vi "initial-Pos-Z.vi"(8 "error in (no error)":errorcluster) -> (0 "error out":errorcluster, 3 "Z position":dbl)   [LabVIEW 2021]
doc: "André Romero - 2023\nandretec@ifsc.usp.br\nIFSC - USP"
uses:
  Global Motors.vi
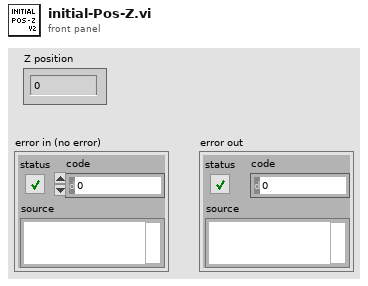
[diagram p1: front panel]
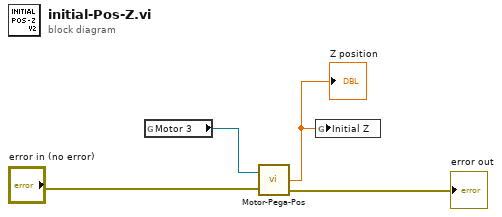
[diagram p0: block diagram]
diagram:
  n1 = global read "Global Motors.vi" "Motor 3"() -> (w4:refnum<k7>)
  n2 = call "Motor-Pega-Pos.vi"("MG17Motor 2"=w4, "error out"="error in (no error)") -> ("pfPosition"=w1:sgl, "error out 2"=→"error out":errorcluster)  [unwired: 1 out]
  "Z position" <- w1
  n3 = global write "Global Motors.vi" "Initial Z"(w1) -> ()
